vi "even sub vi.vi"(9 "String 2":string, 10 "input":dbl, 11 "String":string) -> (3 "String 3":string)   [LabVIEW 2020]
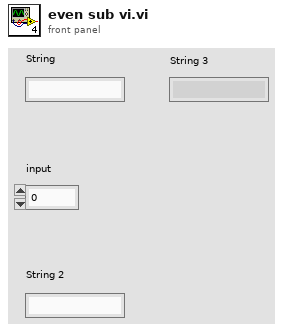
[diagram p1: front panel]
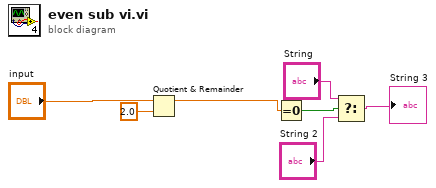
[diagram p0: block diagram]
diagram:
  n1 = Quotient & Remainder(x="input", y=2.0) -> (x-y*floor(x/y)=w1:dbl)  [unwired: 1 out]
  n2 = Equal To 0?(x=w1) -> (x = 0?=w4:bool)
  n3 = Select(t="String", s=w4, f="String 2") -> (s? t:f=→"String 3":string)
